vi "Promotion.vi"() -> (0 "index of element":i32=-1)   [LabVIEW 2014]
panel:
  in  "Cluster":T1
  # "Choose which one you want to promotion to."
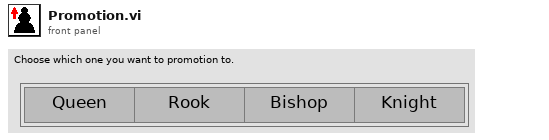
[diagram p1: front panel]
types:
  T1 = cluster{"OK Button":bool, "OK Button 2":bool, "OK Button 3":bool, "OK Button 4":bool}
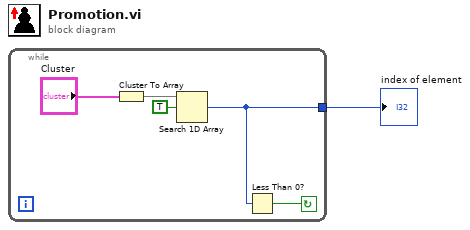
[diagram p0: block diagram]
diagram:
  n1 = while {
    tunnel: [w2] -> w1
    stop <- w3 continue-if-true
    n2 = Cluster To Array(cluster="Cluster") -> (array=w5:bool[])
    n3 = Search 1D Array(1D array=w5, element=TRUE) -> (index of element=w2:i32)  [unwired: 1 in]
    n4 = Less Than 0?(x=w2) -> (x < 0?=w3:bool)
  }
  "index of element" <- w1
